vi "DigitalChartPlotter.vi"(5 "History Size":i32, 7 "Reset?":bool, 10 "Input":u8[](array[numeric])) -> (2 "Digital Data":digitalwaveform(graph))   [LabVIEW 2014]
panel:
  out "f":u64
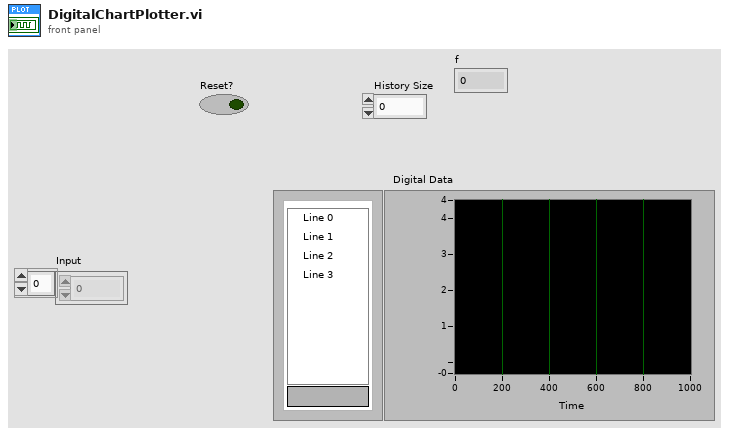
[diagram p1: front panel]
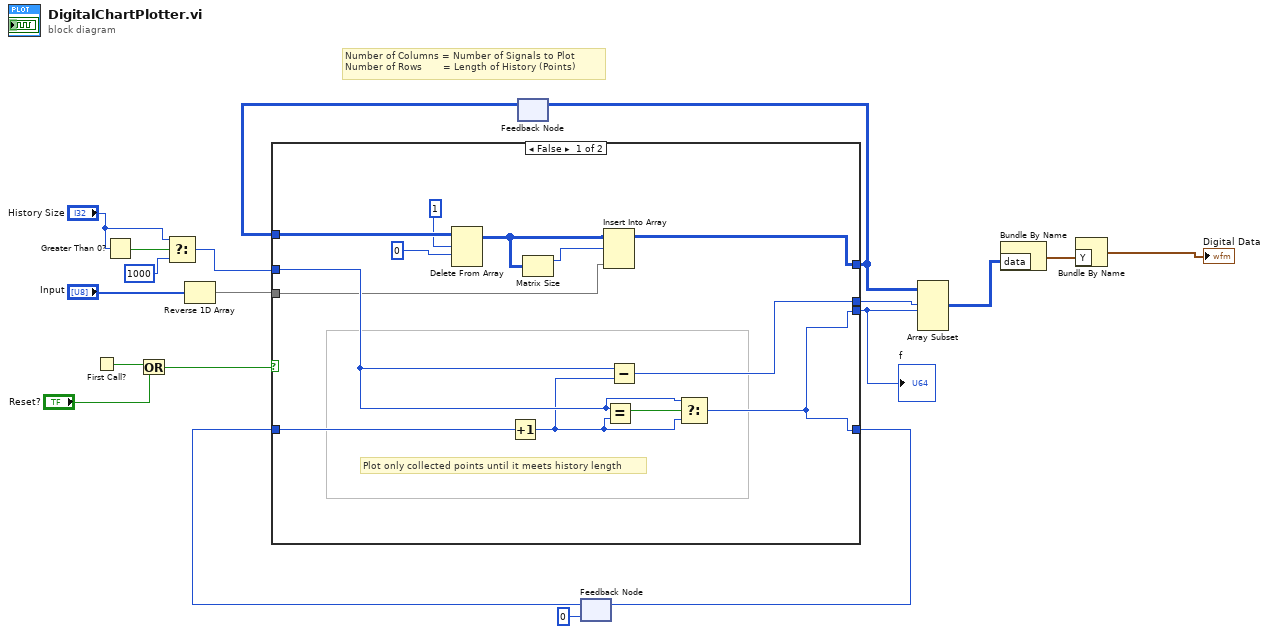
[diagram p0: block diagram]
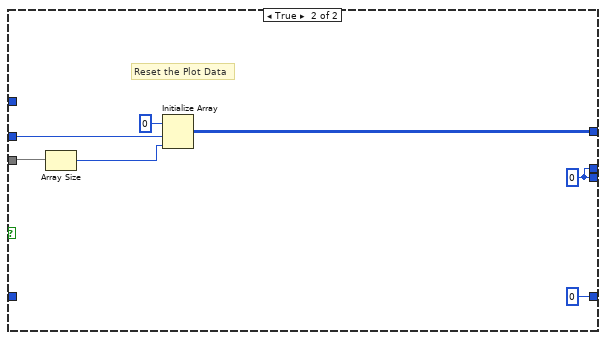
[diagram p2: hidden frame]
diagram:
  # "Number of Columns = Number of Signals to Plot\nNumber of Rows       = Length of History (Points)"
  n1 = First Call?() -> (First Call?: T/F=w18:bool)
  n2 = Greater Than 0?(x="History Size") -> (x > 0?=w15:bool)
  n3 = Or(x=w18, y="Reset?") -> (x .or. y?=w19:bool)
  n4 = Select(t="History Size", s=w15, f=1000) -> (s? t:f=w12:i32)
  n5 = Reverse 1D Array(array="Input") -> (reversed array=w1:u8[])
  n6 = feedback #1() -> (w11:u8[][])  [unwired: 1 in]
  n7 = feedback #2(u64 0) -> (w7:u64)
  n8 = case shown="False" w19 {
    tunnel: w1 -> [w23 w38]
    tunnel: w12 -> [w25 w36]
    tunnel: w11 -> [w32 _]
    tunnel: [w20 w35] -> w5
    tunnel: w7 -> [w29 _]
    tunnel: [w27 u64 0] -> w8
    tunnel: [w27 w33] -> w3
    tunnel: [w26 w33] -> w2
    frame False {
      # "Plot only collected points until it meets history length"
      n9 = Delete From Array(array=w32, length=1, index (row)=0) -> (array with subset deleted=w22:u8[][])  [unwired: 1 in, 1 out]
      n10 = Increment(x=w29) -> (x+1=w24:u64)
      n11 = Matrix Size(0:w22) -> (1:w21:i32)  [unwired: 1 out]
      n12 = Insert Into Array(array=w22, index (row)=w21, new element=w23) -> (w20:u8[][])  [unwired: 1 in]
      n13 = Equal?(x=w25, y=w24) -> (x = y?=w28:bool)
      n14 = Subtract(x=w25, y=w24) -> (x-y=w26:u64)
      n15 = Select(t=w25, s=w28, f=w24) -> (s? t:f=w27:u64)
    }
    frame True {
      w33 = u64 0
      # "Reset the Plot Data"
      n16 = Array Size(array=w38) -> (size(s)=w37:i32)
      n17 = Initialize Array(u8 0 ("element"), w36, w37) -> (w35:u8[][])
    }
  }
  "f" <- w3
  n18 = feedback-in #1(w5) -> ()
  n19 = feedback-in #2(w8) -> ()
  n20 = Array Subset(array=w5, index (row)=w2, length (row)=w3) -> (w4:u8[][])  [unwired: 2 in]
  n21 = Bundle By Name("data"=w4) -> (w10:digitaldata)  [unwired: 1 in]
  n22 = Bundle By Name("Y"=w10) -> (→"Digital Data":digitalwaveform)  [unwired: 1 in]
